vi "e.gate HighSpeedPort Build Online Command.vi"(0 "WriteIndex":i32, 1 "WriteCount":i32, 2 "ValueArray":dbl[](array[numeric]), 3 "ReadIndex":i32, 4 "ReadCount":i32, 5 "error in (no error)":errorcluster, 6 "Configuration  in":T1) -> (12 "Configuration  out":T1, 14 "OffsetWrite":i32, 15 "LengthWrite":i32, 16 "DataWrite":string, 17 "OffsetRead":i32, 18 "LengthRead":i32, 19 "error out":errorcluster)   [LabVIEW 2016]
doc: "This VI is used to code numeric indexes and offsets for HighSpeedPort TCP/IP Online writing to their byte representations."
uses:
  e.gate Configuration.ctl
  e.gate Channel Data.ctl
  e.gate Data Type.ctl
  e.gate Protocol Type.ctl
  e.gate Module  Data.ctl
  e.gateHSP_DLLhandle.ctl
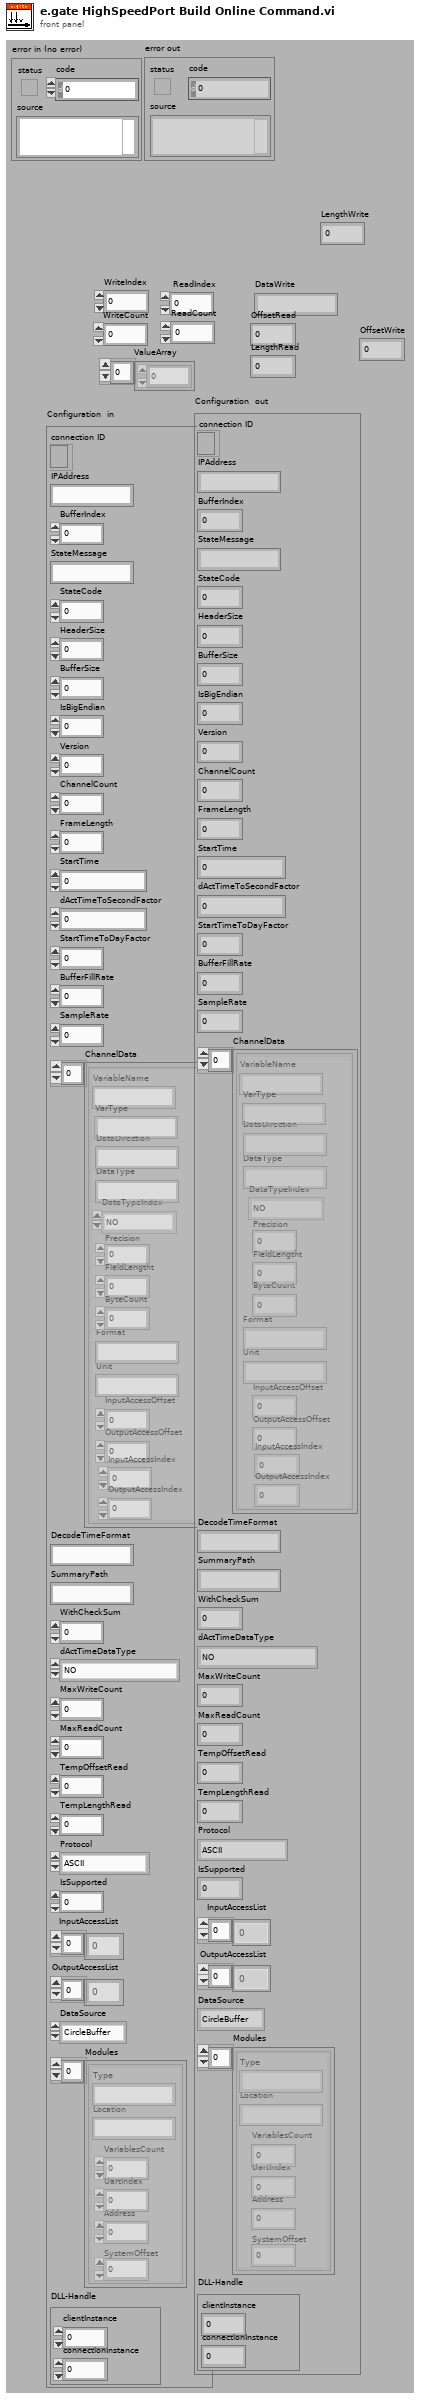
[diagram p1: front panel]
types:
  T1 = typedef "e.gate Configuration.ctl" = cluster{"connection ID":refnum<k5>, "IPAddress":string, "BufferIndex":i32, "StateMessage":string, "StateCode":i8, "HeaderSize":i32, "BufferSize":i32, "IsBigEndian":i32, "Version":i32, "ChannelCount":i32, "FrameLength":i32, "StartTime":dbl, "dActTimeToSecondFactor":dbl, "StartTimeToDayFactor":dbl, "BufferFillRate":dbl, "SampleRate":dbl, "ChannelData":T2[], "DecodeTimeFormat":string, "SummaryPath":string, "WithCheckSum":i32, "dActTimeDataType":T3, "MaxWriteCount":i32, "MaxReadCount":i32, "TempOffsetRead":i32, "TempLengthRead":i32, "Protocol":T4, "IsSupported":i32, "InputAccessList":i32[], "OutputAccessList":i32[], "DataSource":enum16{"CircleBuffer", "test.con Logger", "test.con Archive"}, "Modules":T5[], "DLL-Handle":T6}
  T2 = typedef "e.gate Channel Data.ctl" = cluster{"VariableName":string, "DataDirection":string, "DataType":string, "DataTypeIndex":T3, "Precision":i16, "FieldLengtht":i16, "ByteCount":i32, "Format":string, "Unit":string, "InputAccessOffset":i32, "OutputAccessOffset":i16, "InputAccessIndex":i16, "OutputAccessIndex":i16, "VarType":string}
  T3 = typedef "e.gate Data Type.ctl" = enum16{"NO", "BOOL", "SINT8", "USINT8", "SINT16", "USINT16", "SINT32", "USINT32", "FLOAT", "SET8", "SET16", "SET32", "DOUBLE", "SINT64", "USINT64", "SET64"}
  T4 = typedef "e.gate Protocol Type.ctl" = enum16{"ASCII", "HighspeedPort Online", "HighspeedPort Buffer", "eGateHighspeedPortDLL "}
  T5 = typedef "e.gate Module  Data.ctl" = cluster{"Type":string, "Location":string, "VariablesCount":i16, "UartIndex":i16, "Address":i16, "SystemOffset":i16}
  T6 = typedef "e.gateHSP_DLLhandle.ctl" = cluster{"clientInstance":i32, "connectionInstance":i32}
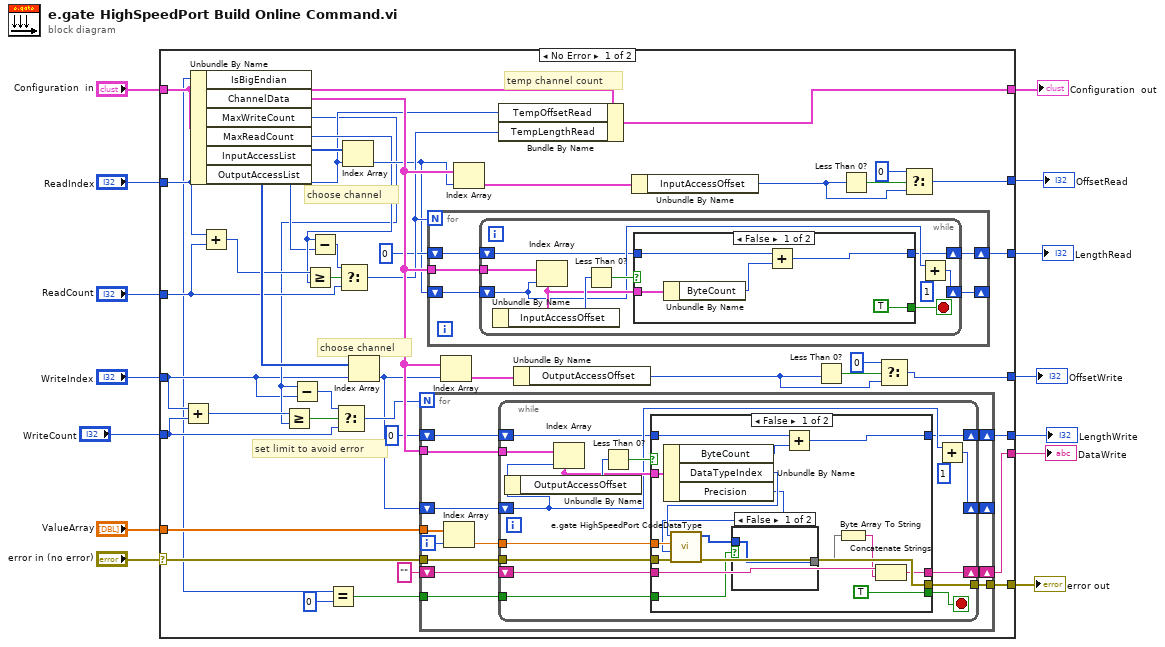
[diagram p0: block diagram]
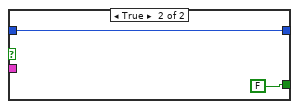
[diagram p2: hidden frame]
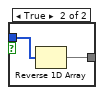
[diagram p3: hidden frame]
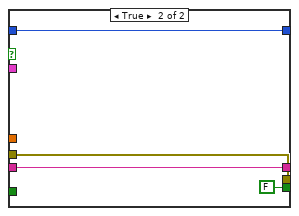
[diagram p4: hidden frame]
diagram:
  n1 = case shown="No Error" "error in (no error)" {
    selector: "error in (no error)" -> [w41 w133]
    tunnel: "Configuration  in" -> [w43 w132]
    tunnel: "ReadIndex" -> [w23 _]
    tunnel: "ReadCount" -> [w27 _]
    tunnel: "WriteCount" -> [w22 _]
    tunnel: "ValueArray" -> [w55 _]
    tunnel: "WriteIndex" -> [w18 _]
    tunnel: [w40 w133] -> w7
    tunnel: [w48 _] -> w6
    tunnel: [w45 _] -> w5
    tunnel: [w34 _] -> w4
    tunnel: [w52 _] -> w3
    tunnel: [w42 w132] -> w2
    tunnel: [w36 _] -> w1
    frame No Error {
      # "choose channel"
      # "choose channel"
      # "set limit to avoid error"
      # "temp channel count"
      n2 = Add(x=w18, y=w22) -> (x+y=w21:i32)
      n3 = Unbundle By Name(w43) -> ("IsBigEndian"=w17:i32, "ChannelData"=w53:T2[], "MaxWriteCount"=w19:i32, "MaxReadCount"=w25:i32, "InputAccessList"=w31:i32[], "OutputAccessList"=w29:i32[])
      n4 = Add(x=w23, y=w27) -> (x+y=w26:i32)
      n5 = Greater Or Equal?(x=w21, y=w19) -> (x >= y?=w38:bool)
      n6 = Subtract(x=w19, y=w18) -> (x-y=w20:i32)
      n7 = Greater Or Equal?(x=w26, y=w25) -> (x >= y?=w39:bool)
      n8 = Subtract(x=w25, y=w23) -> (x-y=w24:i32)
      n9 = Equal?(x=w17, y=0) -> (x = y?=w15:bool)
      n10 = Select(t=w20, s=w38, f=w22) -> (s? t:f=w37:i32)
      n11 = Select(t=w24, s=w39, f=w27) -> (s? t:f=w35:i32)
      n12 = Index Array(array=w31, index=w23) -> (element=w28:i32)
      n13 = Index Array(array=w29, index=w18) -> (element=w30:i32)
      n14 = for {
        N: w37 -> [_]
        tunnel: w55 -> [w92]
        shift-right: [w87] -> w52
        shift-left: "" ("DataWrite") -> [w88]
        tunnel: w53 -> [w90]
        shift-right: [w89] -> _
        shift-left: w30 -> [w86]
        tunnel: w41 -> [w84]
        tunnel: [w83] -> w40
        shift-right: [w81] -> w36
        shift-left: 0 -> [w82]
        tunnel: w15 -> [w80]
        i -> [w91]
        n15 = Index Array(array=w92, index=w91) -> (element=w85:dbl)
        n16 = while {
          tunnel: w90 -> [w102]
          shift-right: [w98] -> w89
          shift-left: w86 -> [w97]
          shift-right: [w105] -> w87
          shift-left: w88 -> [w106]
          tunnel: w85 -> [w103]
          tunnel: w84 -> [w100]
          tunnel: [w99] -> w83
          shift-right: [w95] -> w81
          shift-left: w82 -> [w94]
          tunnel: w80 -> [w93]
          stop <- w104 stop-if-true
          n17 = Index Array(array=w102, index=w97) -> (element=w101:T2)
          n18 = Unbundle By Name(w101) -> ("OutputAccessOffset"=w108:i16)
          n19 = Less Than 0?(x=w108) -> (x < 0?=w107:bool)
          n20 = case shown="False" w107 {
            tunnel: w106 -> [w118 w131]
            tunnel: [w116 w131] -> w105
            tunnel: [TRUE FALSE] -> w104
            tunnel: w103 -> [w123 _]
            tunnel: w101 -> [w122 _]
            tunnel: w100 -> [w120 w129]
            tunnel: [w119 w129] -> w99
            tunnel: [w113 w128] -> w95
            tunnel: w94 -> [w112 w128]
            tunnel: w93 -> [w109 _]
            frame False {
              n21 = Unbundle By Name(w122) -> ("ByteCount"=w114:i32, "DataTypeIndex"=w121:T3, "Precision"=w115:i16)
              n22 = call "e.gate HighSpeedPort CodeDataType.vi"("error in (no error)"=w120, "Precision"=w115, "Value"=w123, "TransferDataType"=w121) -> ("error out"=w119:errorcluster, "Binary data out"=w111:u8[])  [unwired: 6 out]
              n23 = case shown="False" w109 {
                tunnel: w111 -> [w125 w127]
                tunnel: [w125 w126] -> w110
                frame False {
                }
                frame True {
                  n24 = Reverse 1D Array(array=w127) -> (reversed array=w126:u8[])
                }
              }
              n25 = Add(x=w112, y=w114) -> (x+y=w113:i32)
              n26 = Byte Array To String(unsigned byte array=w110) -> (string=w117:string)
              n27 = Concatenate Strings(w118, w117) -> (w116:string)
            }
            frame True {
            }
          }
          n28 = Add(x=w97, y=1) -> (x+y=w98:i32)
        }
      }
      n29 = for {
        N: w35 -> [_]
        tunnel: w53 -> [w62]
        shift-right: [w61] -> w34
        shift-left: 0 -> [w60]
        shift-right: [w58] -> _
        shift-left: w28 -> [w59]
        n30 = while {
          tunnel: w62 -> [w69]
          shift-right: [w67] -> w58
          shift-left: w59 -> [w66]
          shift-right: [w64] -> w61
          shift-left: w60 -> [w63]
          stop <- w70 stop-if-true
          n31 = Index Array(array=w69, index=w66) -> (element=w68:T2)
          n32 = Unbundle By Name(w68) -> ("InputAccessOffset"=w72:i32)
          n33 = Less Than 0?(x=w72) -> (x < 0?=w71:bool)
          n34 = case shown="False" w71 {
            tunnel: [TRUE FALSE] -> w70
            tunnel: w68 -> [w76 _]
            tunnel: [w75 w78] -> w64
            tunnel: w63 -> [w74 w78]
            frame False {
              n35 = Unbundle By Name(w76) -> ("ByteCount"=w73:i32)
              n36 = Add(x=w74, y=w73) -> (x+y=w75:i32)
            }
            frame True {
            }
          }
          n37 = Add(x=w66, y=1) -> (x+y=w67:i32)
        }
      }
      n38 = Index Array(array=w53, index=w30) -> (element=w57:T2)
      n39 = Index Array(array=w53, index=w28) -> (element=w56:T2)
      n40 = Bundle By Name(cluster=w43, "TempOffsetRead"=w23, "TempLengthRead"=w35) -> (w42:T1)
      n41 = Unbundle By Name(w57) -> ("OutputAccessOffset"=w49:i16)
      n42 = Unbundle By Name(w56) -> ("InputAccessOffset"=w44:i32)
      n43 = Less Than 0?(x=w49) -> (x < 0?=w50:bool)
      n44 = Less Than 0?(x=w44) -> (x < 0?=w47:bool)
      n45 = Select(t=i16 0, s=w50, f=w49) -> (s? t:f=w48:i16)
      n46 = Select(t=i16 0, s=w47, f=w44) -> (s? t:f=w45:i32)
    }
    frame Error {
    }
  }
  "Configuration  out" <- w2
  "error out" <- w7
  "OffsetWrite" <- w6
  "DataWrite" <- w3
  "OffsetRead" <- w5
  "LengthRead" <- w4
  "LengthWrite" <- w1
